vi "Write.vi"(4 "size (unlimited)":i32, 7 "timeout in ms (-1)":i32=-1, 9 "last element? (F)":bool, 10 "element":T1, 11 "element valid? (T)":bool=TRUE) -> (2 "channel":T2, 3 "count":i32, 5 "timed out?":bool)   [LabVIEW 2017, in "Stream-t'WPI_EncoderType.ctl'.lvlib"]
doc: "Writes an element to a Stream channel. The endpoint waits if the channel is full."
uses:
  <extravilib>/ChannelInstances/Stream-t'WPI_EncoderType.ctl'.lvlib
  <extravilib>/ChannelInstances/Stream-t'WPI_EncoderType.ctl'/)Channel.ctl
  <vilib>/Rock Robotics/WPI/Encoder/WPI_EncoderType.ctl
  <extravilib>/ChannelInstances/Stream-t'WPI_EncoderType.ctl'/Endpoint.vi
  <resource>/ChannelSupport/_ChannelSupport/WaitIfNeeded.vi
  <extravilib>/ChannelInstances/Stream-t'WPI_EncoderType.ctl'/)Channel.vi
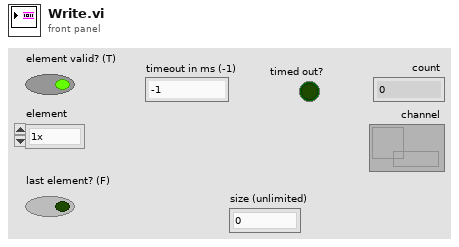
[diagram p1: front panel]
types:
  T1 = typedef "WPI_EncoderType.ctl" = enum16{"1x", "2x", "4x"}
  T2 = typedef "Stream-t'WPI_EncoderType.ctl'.lvlib/)Channel.ctl" = refnum<queue>
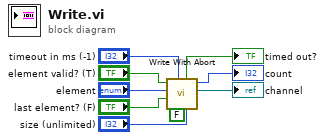
[diagram p0: block diagram]
diagram:
  n1 = call <extravilib>:"Write With Abort.vi"("size (unlimited)"="size (unlimited)", "abort"=FALSE, "timeout in ms (-1)"="timeout in ms (-1)", "last element? (F)"="last element? (F)", "element"="element", "element valid? (T)"="element valid? (T)") -> ("channel"=→"channel":T2, "count"=→"count":i32, "timed out?"=→"timed out?":bool)  [unwired: 2 in, 1 out]
